vi "test Modify Alias and Endpont.vi"(8 "error in (no error)":errorcluster, 11 "TestCase in":refnum<class "Switch Scripting Unit Tests.lvclass">) -> (0 "error out":errorcluster, 3 "TestCase out":refnum<class "Switch Scripting Unit Tests.lvclass">)   [LabVIEW 2017, in "Switch Scripting Unit Tests.lvclass"]
uses:
  Switch Scripting Unit Tests.lvclass
  Switch Scripting Unit Tests.lvclass/Switch Scripting Unit Tests.ctl
  <vilib>/addons/_JKI Toolkits/VI Tester/TestCase.llb/TestCase.lvclass
  Switch Scripting.lvlib
  C:/Program Files (x86)/National Instruments/LabVIEW 2017/vi.lib/addons/_JKI Toolkits/VI Tester/TestCase.llb/TestCase.lvclass
panel:
  in  "Save?":bool
  out "Output Filename":string
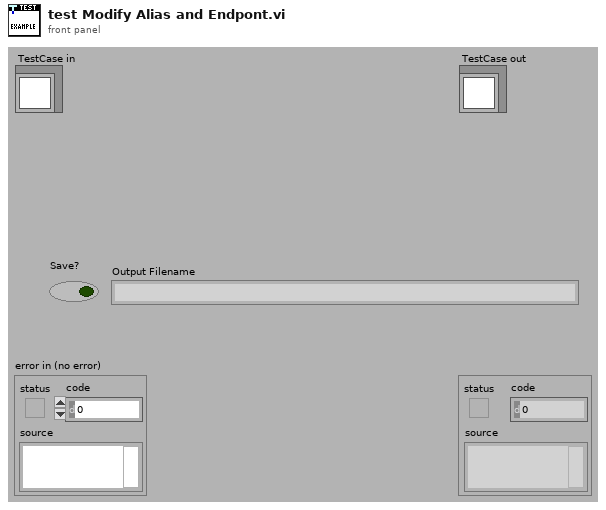
[diagram p1: front panel]
types:
  T1 = typedef "Custom Device API.lvlib/Custom Device Item Ref.ctl" = u64
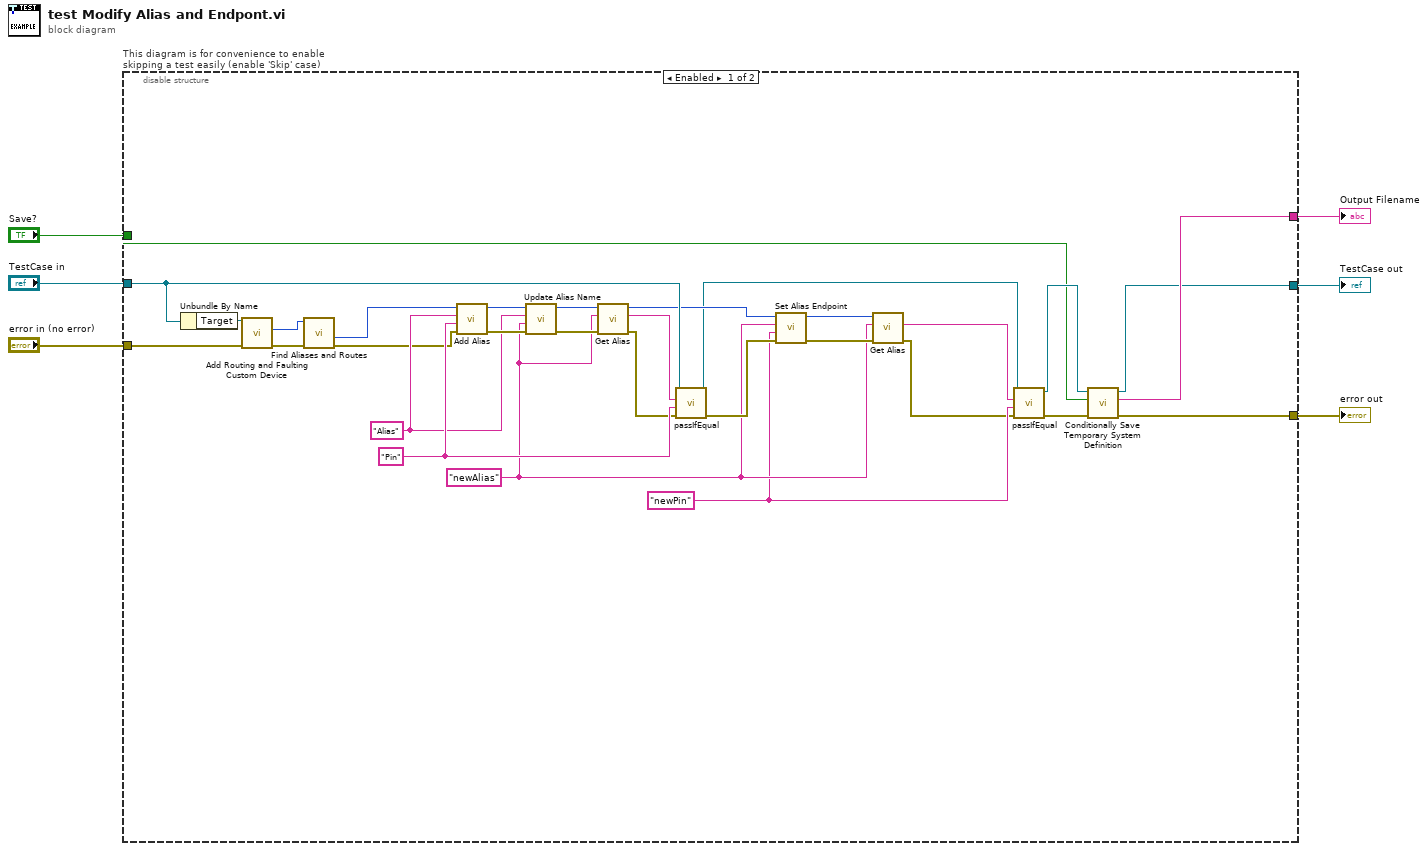
[diagram p0: block diagram]
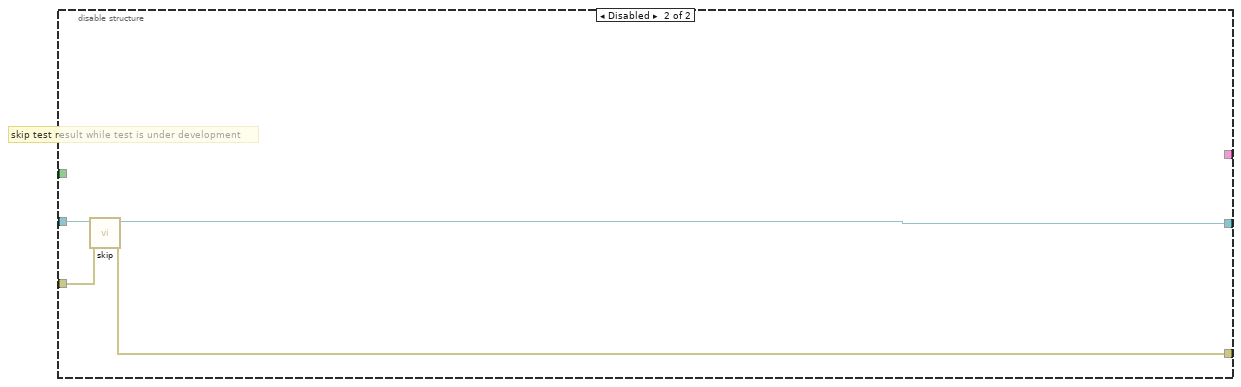
[diagram p2: hidden frame]
diagram:
  n1 = disable-structure "This diagram is for convenience to enable skipping a test easily (enable 'Skip' case)" shown="Enabled" {
    disable-tunnel: "TestCase in" -> [w31 w40]
    disable-tunnel: [w34 w38] -> w3
    disable-tunnel: [w35 w39] -> w5
    disable-tunnel: "error in (no error)" -> [w32 w37]
    disable-tunnel: [w36 _] -> w2
    disable-tunnel: "Save?" -> [w10 _]
    frame Enabled {
      w12 = "newPin" ("Pin")
      w15 = "newAlias" ("Alias")
      w28 = "Pin" ("Pin")
      w20 = "Alias" ("Alias")
      n2 = Unbundle By Name(w31) -> ("Target"=w33:refnum<k24>)
      n3 = call "Add Routing and Faulting Custom Device.vi"("error in (no error)"=w32, "Target in"=w33) -> ("error out"=w30:errorcluster, "RaF CD Ref"=w8:T1)  [unwired: 7 in, 1 out]
      n4 = call "Find Aliases and Routes.vi"("error in (no error)"=w30, "RaF CD Ref in"=w8) -> ("error out"=w9:errorcluster, "Aliases Section Ref"=w7:T1)  [unwired: 6 in, 2 out]
      n5 = call "Add Alias.vi"("error in (no error)"=w9, "Endpont"=w28, "Alias"=w20, "Aliases Ref in"=w7) -> ("error out"=w22:errorcluster, "Aliases Ref out"=w24:T1)  [unwired: 6 in]
      n6 = call "Update Alias Name.vi"("error in (no error)"=w22, "New Alias name"=w15, "Alias"=w20, "Aliases Ref in"=w24) -> ("error out"=w21:errorcluster, "Aliases Ref out"=w23:T1)  [unwired: 6 in]
      n7 = call "Get Alias.vi"("error in (no error)"=w21, "Alias"=w15, "Aliases Ref in"=w23) -> ("error out"=w27:errorcluster, "Endpont"=w29:string, "Aliases Ref out"=w19:T1)  [unwired: 6 in]
      n8 = call-dynamic "passIfEqual.vi"("error in (no error)"=w27, "y"=w28, "x"=w29, "TestCase in"=w31) -> ("error out"=w18:errorcluster, "TestCase out"=w14:refnum<class "Switch Scripting Unit Tests.lvclass">)  [unwired: 6 in]
      n9 = call "Set Alias Endpoint.vi"("error in (no error)"=w18, "New Endpont"=w12, "Alias"=w15, "Aliases Ref in"=w19) -> ("error out"=w16:errorcluster, "Aliases Ref out"=w17:T1)  [unwired: 6 in]
      n10 = call "Get Alias.vi"("error in (no error)"=w16, "Alias"=w15, "Aliases Ref in"=w17) -> ("error out"=w11:errorcluster, "Endpont"=w13:string)  [unwired: 6 in, 1 out]
      n11 = call-dynamic "passIfEqual.vi"("error in (no error)"=w11, "y"=w12, "x"=w13, "TestCase in"=w14) -> ("error out"=w25:errorcluster, "TestCase out"=w26:refnum<class "Switch Scripting Unit Tests.lvclass">)  [unwired: 6 in]
      n12 = call "Conditionally Save Temporary System Definition.vi"("error in (no error)"=w25, "Save?"=w10, "Test Case"=w26) -> ("error out"=w35:errorcluster, "filename"=w36:string, "Test Case"=w34:refnum<class "Switch Scripting Unit Tests.lvclass">)  [unwired: 6 in]
    }
    frame Disabled {
      # "skip test result while test is under development"
      n13 = call <vilib>:"skip.vi"("error in (no error)"=w37, "TestCase in"=w40) -> ("error out"=w39:errorcluster, "TestCase out"=w38:refnum<class "Switch Scripting Unit Tests.lvclass">)  [unwired: 8 in]
    }
  }
  "error out" <- w5
  "TestCase out" <- w3
  "Output Filename" <- w2
